vi "PH_Cont-601k_PSU.set Voltage.vi"(0 "VI in":refnum<vi>, 2 "Voltage [V]":u16, 5 "error in (no error)":errorcluster) -> (14 "VI out":refnum<vi>, 16 "Voltage changed":bool, 19 "error out":errorcluster)   [LabVIEW 2014, in "PH_Cont-601k_PSU.lvlib"]
doc: "Thios VI sets the incoming voltage to own attributes, indivcates it at the related GUI element and renews the DIM service."
uses:
  PH_Cont-601k_PSU.lvlib
  PH_Basics/PH_Common/PH_Common.lvlib
  CSlibraries-extern/DimLVEvent/LVDimInterface/LVDimInterface.lvlib
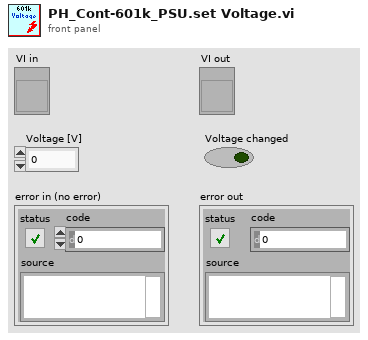
[diagram p1: front panel]
types:
  T1 = typedef "PH_Cont-601k_PSU.lvlib/PH_Cont-601k_PSU.i attribute.ctl" = cluster{"GUI Refs":T2, "Interlock":bool, "Service ID applied Voltage":i32, "Device Settings":cluster{"Configuration":T3, "Flash Interval [s]":dbl, "Mode":T4, "Voltage [V]":u16, "Charge":bool, "VISA resource name":refnum<visa-resource-name>}, "Readyness":T5, "Information":cluster{"VISA resource name":refnum<visa-resource-name>, "Tagname Power On":string, "Interlock":cluster{"Instance":string, "Tagname":string}, "Limits [V]":cluster{"Lower":dbl, "Upper":dbl}, "Tagname PSU On":string}, "R2S":bool, "Charge is allowed":bool}
  T2 = typedef "PH_Cont-601k_PSU.lvlib/PH_Cont-601k_PSU.GUI Refs.ctl" = cluster{"Power On":refnum<vi>, "Hard- and Software":refnum<vi>, "Device Status":refnum<vi>, "Device Error":refnum<vi>, "Configuration":refnum<vi>, "Flash Interval [s]":refnum<vi>, "Interlock":refnum<vi>, "Interlock Indicator":refnum<vi>, "Voltage [V]":refnum<vi>, "Readyness":refnum<vi>, "Mode":refnum<vi>, "Reset Error":refnum<vi>, "Expert working":refnum<vi>, "Charge":refnum<vi>, "PSU On":refnum<vi>}
  T3 = typedef "PH_Cont-601k_PSU.lvlib/PH_Cont-601k_PSU.Configuration.ctl" = u16
  T4 = typedef "PH_Cont-601k_PSU.lvlib/PH_Cont-601k_PSU.Mode.ctl" = enum32{"STOP", "STANDBY", "READY", "EMISSION", "ERROR"}
  T5 = typedef "PH_Cont-601k_PSU.lvlib/PH_Cont-601k_PSU.Readyness.ctl" = cluster{"Program":T6, "Device":T7}
  T6 = typedef "PH_Cont-601k_PSU.lvlib/PH_Cont-601k_PSU.Readyness Program.ctl" = enum32{"OFF", "POWER", "INTERLOCK"}
  T7 = typedef "PH_Cont-601k_PSU.lvlib/PH_Cont-601k_PSU.Readyness Device.ctl" = enum32{"OFF", "CONNECTING", "CONNECTED", "OPERATING", "EOC", "ERROR"}
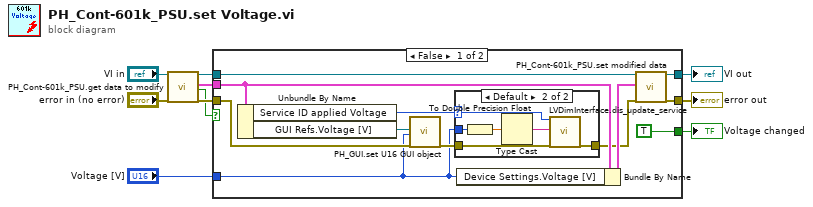
[diagram p0: block diagram]
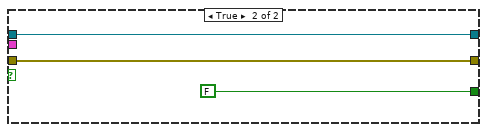
[diagram p3: hidden frame]
diagram:
  n1 = call "PH_Cont-601k_PSU.get data to modify.vi"("i ref in"="VI in", "error in (no error)"="error in (no error)") -> ("i ref out"=w4:refnum<vi>, "i attribute"=w2:T1, "timed out"=w1:bool, "error out"=w5:errorcluster)  [unwired: 14 in]
  n2 = case shown="False" w1 {
    tunnel: [w19 w31] -> w6
    tunnel: w5 -> [w17 w31]
    tunnel: w4 -> [w18 w32]
    tunnel: [w20 w32] -> w3
    tunnel: w2 -> [w16 _]
    tunnel: "Voltage [V]" -> [w12 _]
    tunnel: [TRUE FALSE] -> w10
    frame False {
      n3 = Unbundle By Name(w16) -> ("Service ID applied Voltage"=w11:i32, "GUI Refs.Voltage [V]"=w21:refnum<vi>)
      n4 = call "PH_GUI.set U16 GUI object.vi"("U16 Ref"=w21, "Value"=w12, "error in (no error)"=w17) -> ("error out"=w14:errorcluster)  [unwired: 16 in]
      n5 = case shown="Default" w11 {
        selector: w11 -> [_ w27]
        tunnel: [w23 w28] -> w13
        tunnel: w14 -> [w23 w29]
        tunnel: w12 -> [_ w25]
        frame -1 {
        }
        frame Default {
          n6 = To Double Precision Float(number=w25) -> (double precision float=w24:dbl)
          n7 = Type Cast(x=w24) -> (*(type *) &x=w26:string)  [unwired: 1 in]
          n8 = call "LVDimInterface.dis_update_service.vi"("my_serviceID"=w27, "data"=w26, "error in (no error)"=w29) -> ("error out"=w28:errorcluster)  [unwired: 14 in, 2 out]
        }
      }
      n9 = Bundle By Name(cluster=w16, "Device Settings.Voltage [V]"=w12) -> (w22:T1)
      n10 = call "PH_Cont-601k_PSU.set modified data.vi"("i ref in"=w18, "i attribute"=w22, "error in (no error)"=w13) -> ("i ref out"=w20:refnum<vi>, "error out"=w19:errorcluster)  [unwired: 15 in]
    }
    frame True {
    }
  }
  "Voltage changed" <- w10
  "error out" <- w6
  "VI out" <- w3
